vi "payload-1D-2D.vi"(4 "Array":bool[](array[boolean])) -> (1 "Array 2":bool[][](array[boolean]))   [LabVIEW 2015]
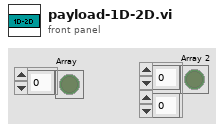
[diagram p1: front panel]
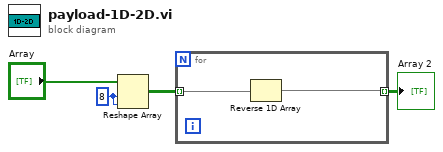
[diagram p0: block diagram]
diagram:
  w4 = 8 ("dimension size")
  n1 = Reshape Array("Array", w4, w4) -> (w2:bool[][])
  n2 = for {
    tunnel: w2 -> [w6] mode=indexing
    tunnel: [w5] -> w1 mode=indexing
    n3 = Reverse 1D Array(array=w6) -> (reversed array=w5:bool[])
  }
  "Array 2" <- w1
